vi "digitalInput.vi"(3 "error in":errorcluster, 4 "Channel":u16(ring) items=["FIO0", "FIO1", "FIO2", "FIO3", "FIO4", "FIO5", "FIO6", "FIO7", "EIO0", "EIO1", "EIO2", "EIO3", "EIO4", "EIO5", "EIO6", "EIO7", "CIO0", "CIO1", "CIO2", "CIO3", "MIO0", "MIO1", "MIO2"], 5 "Handle In":i32) -> (0 "error out":errorcluster, 1 "State":i32, 2 "Handle Out":i32)   [LabVIEW 2021]
panel:
  # "inputs"
  # "outputs"
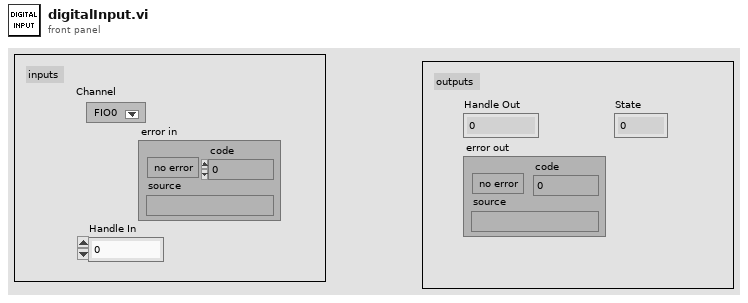
[diagram p1: front panel]
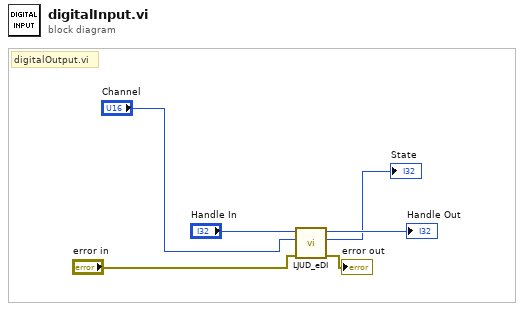
[diagram p0: block diagram]
diagram:
  # "digitalOutput.vi"
  n1 = call <vilib>:"LJUD_eDI.vi"("error in"="error in", "Channel"="Channel", "Handle In"="Handle In") -> ("error out"=→"error out":errorcluster, "State"=→"State":i32, "Handle Out"=→"Handle Out":i32)  [unwired: 6 in]
